vi "Array to Offset and Multiplier.vi"(1 "Array":dbl[](array[numeric])) -> (0 "Offset and Multiplier":T1)   [LabVIEW 2016, in "graph_utilities.lvclass"]
doc: "Given an array, calculate an Offset and Multiplier"
uses:
  graph_utilities.lvclass
  <vilib>/Utility/miscctls.llb/LVOffsetAndMultiplierTypeDef.ctl
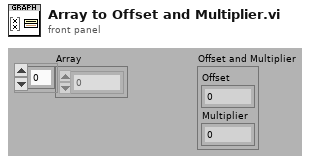
[diagram p1: front panel]
types:
  T1 = typedef "LVOffsetAndMultiplierTypeDef.ctl" = cluster{"Offset":dbl, "Multiplier":dbl}
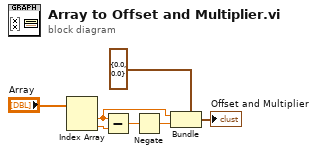
[diagram p0: block diagram]
diagram:
  n1 = Index Array(array="Array") -> (element #1=w7:dbl, element #2=w4:dbl)  [unwired: 2 in]
  n2 = Subtract(x=w7, y=w4) -> (x-y=w5:dbl)
  n3 = Negate(x=w5) -> (-x=w6:dbl)
  n4 = Bundle(cluster=T1 {"Offset"=0.0, "Multiplier"=0.0} ("X Scale.Offset and Multiplier"), "Offset"=w7, "Multiplier"=w6) -> (→"Offset and Multiplier":T1)
